vi "HPPC_Test.vi"() -> ()   [LabVIEW 2020]
panel:
  in  "FilePath":path=path "C:/Users/ga11/Desktop/VI/results/3PtestCharge.lvm" caption="Filename"
  in  "P task error in":errorcluster
  in  "Pulse C-rate":dbl format="%#.6g"
  in  "Capacity (Ah)":dbl format="%#.6g"
  in  "Parallel Task in":refnum<k21>
  out "Relay error out":errorcluster
  in  "Battery Select":i32
  in  "NHR error in":errorcluster caption="error in (no error)"
  in  "NHR VISA":refnum<visa-resource-name>
  in  "task error in":errorcluster
  in  "Relay Task":refnum<k21>
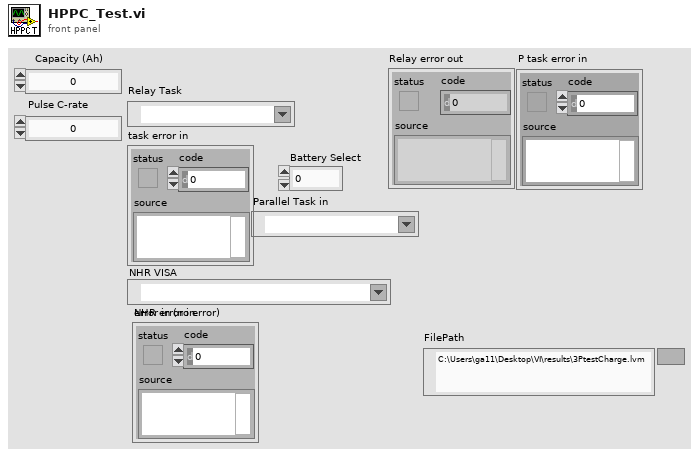
[diagram p1: front panel]
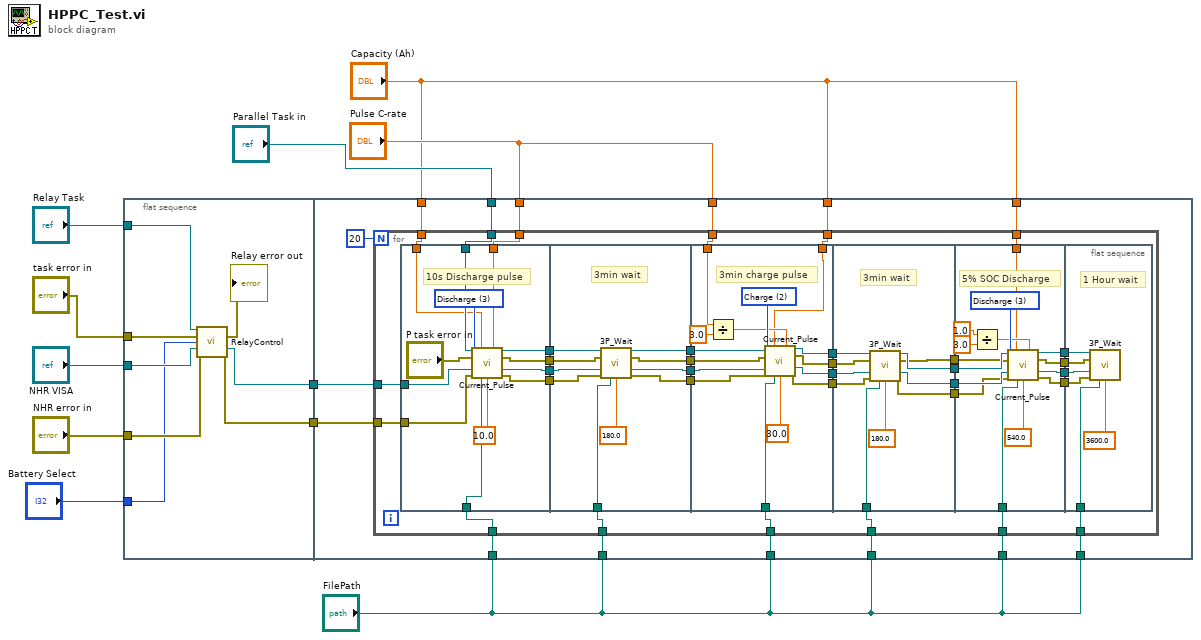
[diagram p0: block diagram]
diagram:
  n1 = flat-sequence {
    tunnel: "Relay Task" -> [w19]
    tunnel: "task error in" -> [w18]
    tunnel: "NHR VISA" -> [w17]
    tunnel: "NHR error in" -> [w16]
    tunnel: "Battery Select" -> [w15]
    tunnel: [w13] -> w5
    tunnel: [w12] -> w4
    tunnel: "Pulse C-rate" -> [w33]
    tunnel: "FilePath" -> [w32]
    tunnel: "Parallel Task in" -> [w31]
    tunnel: w5 -> [w30]
    tunnel: w4 -> [w29]
    tunnel: "FilePath" -> [w28]
    tunnel: "FilePath" -> [w27]
    tunnel: "Pulse C-rate" -> [w26]
    tunnel: "Capacity (Ah)" -> [w25]
    tunnel: "Capacity (Ah)" -> [w24]
    tunnel: "FilePath" -> [w23]
    tunnel: "Capacity (Ah)" -> [w22]
    tunnel: "FilePath" -> [w21]
    tunnel: "FilePath" -> [w20]
    frame #0 {
      n2 = call "RelayControl.vi"("Relay Task"=w19, "error in"=w18, "Battery Select (0: Off)"=w15, "NHR VISA"=w17, "NHR error in"=w16) -> ("error out"=→"Relay error out":errorcluster, "NHR Visa out"=w13:refnum<visa-resource-name>, "NHR error out"=w12:errorcluster)  [unwired: 8 in]
    }
    frame #1 {
      n3 = for {
        N: 20 -> [_]
        tunnel: w33 -> [w68]
        tunnel: w32 -> [w67]
        tunnel: w31 -> [w66]
        tunnel: w30 -> [w65]
        tunnel: w29 -> [w64]
        tunnel: w28 -> [w63]
        tunnel: w27 -> [w62]
        tunnel: w26 -> [w61]
        tunnel: w25 -> [w60]
        tunnel: w24 -> [w59]
        tunnel: w23 -> [w58]
        tunnel: w22 -> [w57]
        tunnel: w21 -> [w56]
        tunnel: w20 -> [w55]
        n4 = flat-sequence {
          tunnel: w68 -> [w80]
          tunnel: w67 -> [w79]
          tunnel: w66 -> [w78]
          tunnel: w65 -> [w77]
          tunnel: w64 -> [w76]
          tunnel: w60 -> [w73]
          tunnel: [w72] -> w54
          tunnel: [w71] -> w53
          tunnel: [w70] -> w52
          tunnel: [w69] -> w51
          tunnel: w63 -> [w90]
          tunnel: w54 -> [w89]
          tunnel: w53 -> [w88]
          tunnel: w52 -> [w87]
          tunnel: w51 -> [w86]
          tunnel: [w85] -> w50
          tunnel: [w84] -> w49
          tunnel: [w83] -> w48
          tunnel: [w82] -> w47
          tunnel: w62 -> [w104]
          tunnel: w61 -> [w102]
          tunnel: w59 -> [w100]
          tunnel: w50 -> [w99]
          tunnel: w49 -> [w98]
          tunnel: w48 -> [w97]
          tunnel: w47 -> [w96]
          tunnel: [w95] -> w46
          tunnel: [w94] -> w45
          tunnel: [w93] -> w44
          tunnel: [w92] -> w43
          tunnel: w58 -> [w115]
          tunnel: w46 -> [w114]
          tunnel: w45 -> [w113]
          tunnel: w44 -> [w112]
          tunnel: w43 -> [w111]
          tunnel: [w110] -> w42
          tunnel: [w109] -> w41
          tunnel: [w108] -> w40
          tunnel: [w107] -> w39
          tunnel: w57 -> [w126]
          tunnel: w56 -> [w125]
          tunnel: w42 -> [w124]
          tunnel: w41 -> [w123]
          tunnel: w40 -> [w122]
          tunnel: w39 -> [w121]
          tunnel: [w120] -> w38
          tunnel: [w119] -> w37
          tunnel: [w118] -> w36
          tunnel: [w117] -> w35
          tunnel: w55 -> [w136]
          tunnel: w38 -> [w135]
          tunnel: w37 -> [w134]
          tunnel: w36 -> [w133]
          tunnel: w35 -> [w132]
          frame #0 {
            w75 = 3 items=["Off", "Standby", "Charge", "Discharge", "Battery"] ("Mode (2: Charge, 3: Discharge)")
            # "10s Discharge pulse"
            n5 = call "Current_Pulse.vi"("Parallel Task in"=w78, "Capacity (Ah)"=w73, "C rate Setpoint"=w80, "P task error in"="P task error in", "Mode (2: Charge, 3: Discharge)"=w75, "NHR VISA in"=w77, "NHR error in"=w76, "FilePath"=w79, "Wait time (s)"=10.0) -> ("parallel task out"=w72:refnum<k21>, "parallel task error out"=w71:errorcluster, "VISA resource name out"=w70:refnum<visa-resource-name>, "NHR error out"=w69:errorcluster)  [unwired: 3 in]
          }
          frame #1 {
            # "3min wait"
            n6 = call "3P_Wait.vi"("Parallel Task in"=w89, "P task error in"=w88, "NHR VISA in"=w87, "NHR error in"=w86, "Wait Filepath"=w90, "Wait time"=180.0) -> ("parallel task out"=w85:refnum<k21>, "parallel task error out"=w84:errorcluster, "NHR Visa Out"=w83:refnum<visa-resource-name>, "NHR error out"=w82:errorcluster)  [unwired: 5 in, 1 out]
          }
          frame #2 {
            w106 = 2 items=["Off", "Standby", "Charge", "Discharge", "Battery"] ("Mode (2: Charge, 3: Discharge)")
            # "3min charge pulse"
            n7 = Divide(x=w102, y=3.0) -> (x/y=w101:dbl)
            n8 = call "Current_Pulse.vi"("Parallel Task in"=w99, "Capacity (Ah)"=w100, "C rate Setpoint"=w101, "P task error in"=w98, "Mode (2: Charge, 3: Discharge)"=w106, "NHR VISA in"=w97, "NHR error in"=w96, "FilePath"=w104, "Wait time (s)"=30.0) -> ("parallel task out"=w95:refnum<k21>, "parallel task error out"=w94:errorcluster, "VISA resource name out"=w93:refnum<visa-resource-name>, "NHR error out"=w92:errorcluster)  [unwired: 3 in]
          }
          frame #3 {
            # "3min wait"
            n9 = call "3P_Wait.vi"("Parallel Task in"=w114, "P task error in"=w113, "NHR VISA in"=w112, "NHR error in"=w111, "Wait Filepath"=w115, "Wait time"=180.0) -> ("parallel task out"=w110:refnum<k21>, "parallel task error out"=w109:errorcluster, "NHR Visa Out"=w108:refnum<visa-resource-name>, "NHR error out"=w107:errorcluster)  [unwired: 5 in, 1 out]
          }
          frame #4 {
            w131 = 3 items=["Off", "Standby", "Charge", "Discharge", "Battery"] ("Mode (2: Charge, 3: Discharge)")
            # "5% SOC Discharge"
            n10 = Divide(x=1.0, y=3.0) -> (x/y=w128:dbl)
            n11 = call "Current_Pulse.vi"("Parallel Task in"=w124, "Capacity (Ah)"=w126, "C rate Setpoint"=w128, "P task error in"=w123, "Mode (2: Charge, 3: Discharge)"=w131, "NHR VISA in"=w122, "NHR error in"=w121, "FilePath"=w125, "Wait time (s)"=540.0) -> ("parallel task out"=w120:refnum<k21>, "parallel task error out"=w119:errorcluster, "VISA resource name out"=w118:refnum<visa-resource-name>, "NHR error out"=w117:errorcluster)  [unwired: 3 in]
          }
          frame #5 {
            # "1 Hour wait"
            n12 = call "3P_Wait.vi"("Parallel Task in"=w135, "P task error in"=w134, "NHR VISA in"=w133, "NHR error in"=w132, "Wait Filepath"=w136, "Wait time"=3600.0) -> ()  [unwired: 5 in, 5 out]
          }
        }
      }
    }
  }
